vi "square_source.vi"(2 "pause":bool, 3 "square_control":T1) -> (0 "Terminate?":bool, 1 "output_signal":dbl)   [LabVIEW 2014]
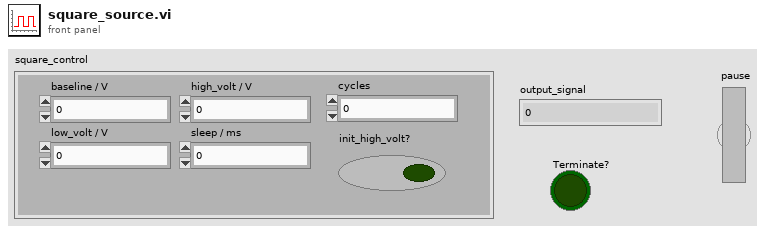
[diagram p1: front panel]
types:
  T1 = cluster{"baseline / V":dbl, "low_volt / V":dbl, "high_volt / V":dbl, "sleep / ms":u32, "init_high_volt?":bool, "cycles":u32}
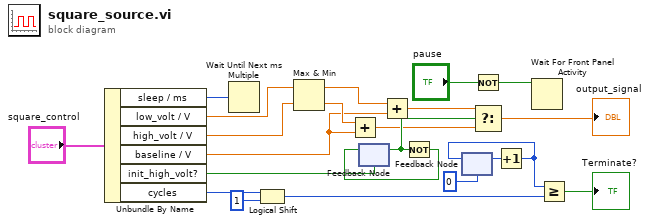
[diagram p0: block diagram]
diagram:
  n1 = Unbundle By Name("square_control") -> ("sleep / ms"=w13:u32, "low_volt / V"=w12:dbl, "high_volt / V"=w11:dbl, "baseline / V"=w10:dbl, "init_high_volt?"=w14:bool, "cycles"=w9:u32)
  n2 = Wait Until Next ms Multiple(millisecond multiple=w13) -> ()  [unwired: 1 out]
  n3 = Logical Shift(y=w9, x=u32 1) -> (x << y=w6:u32)
  n4 = Max & Min(x=w12, y=w11) -> (max(x,y)=w20:dbl, min(x,y)=w19:dbl)
  n5 = Add(x=w19, y=w10) -> (x+y=w18:dbl)
  n6 = feedback #1(w14) -> (w22:bool)
  n7 = Add(x=w20, y=w10) -> (x+y=w17:dbl)
  n8 = Not(x=w22) -> (.not. x?=w21:bool)
  n9 = feedback-in #1(w21) -> ()
  n10 = feedback #2(0) -> (w5:i32)
  n11 = Not(x="pause") -> (.not. x?=w2:bool)
  n12 = Select(t=w17, s=w22, f=w18) -> (s? t:f=→"output_signal":dbl)
  n13 = Increment(x=w5) -> (x+1=w1:i32)
  n14 = feedback-in #2(w1) -> ()
  n15 = Wait For Front Panel Activity(3:w2) -> ()  [unwired: 2 in, 1 out]
  n16 = Greater Or Equal?(x=w1, y=w6) -> (x >= y?=→"Terminate?":bool)
